vi "Find Object Items.vi"   [LabVIEW 2015, in "JSONtext.lvlib"]
uses:
  JSONtext.lvlib
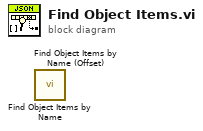
[diagram p0: block diagram]
diagram:
  n1 = call "Find Object Items by Name.vi"() -> ()  [unwired: 9 in, 3 out]
  n2 = call "Find Object Items by Name (Offset).vi"() -> ()  [unwired: 9 in, 3 out]
